vi "Average Grayscale of Line.vi"(8 "nPoints":i32, 9 "offset":i32, 10 "row":i32, 11 "24-bit pixmap in":u32[][](array[numeric])) -> (2 "average grayscale":sgl, 3 "24-bit pixmap out":u32[][](array[numeric]))   [LabVIEW 2020, in "lv_icon.lvlib"]
doc: "Find the average grayscale value along one row of a 24-bit pixmap. Uses the luminance formula:\n\nGrayscale = 0.2126 R + 0.7152 G + 0.0722 B\n\nWhere R, G, and B are the red, green, and blue intensities, respectively."
uses:
  resource/plugins/lv_icon.lvlib
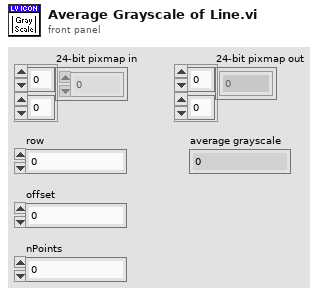
[diagram p1: front panel]
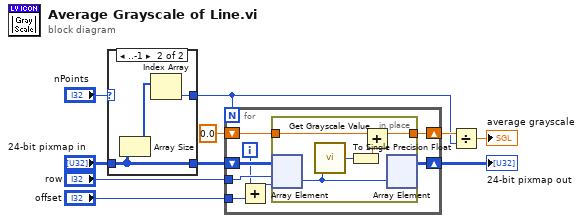
[diagram p0: block diagram]
diagram:
  n1 = case shown="..-1" "nPoints" {
    selector: "nPoints" -> [w12 _]
    tunnel: [w12 w14] -> w4
    tunnel: "24-bit pixmap in" -> [w11 w13]
    tunnel: [w11 w13] -> w2
    frame 0.. {
    }
    frame ..-1 {
      n2 = Array Size(array=w13) -> (size(s)=w15:i32[])
      n3 = Index Array(array=w15) -> (element=w14:i32)  [unwired: 1 in]
    }
  }
  n4 = for {
    N: w4 -> [_]
    tunnel: "row" -> [w22]
    shift-right: [w19] -> w9
    shift-left: sgl 0.0 ("single precision float") -> [w20]
    shift-right: [w18] -> w10
    shift-left: w2 -> [w23]
    tunnel: "offset" -> [w16]
    i -> [w17]
    n5 = Add(x=w17, y=w16) -> (x+y=w21:i32)
    n6 = in-place {
      in-place-border: w20 -> [w26]
      in-place-border: [w24] -> w19
      n7 = in-place-array #1(w23, w22, w21) -> (w28:u32)
      n8 = call "Get Grayscale Value.vi"("input color"=w28) -> ("grayscale value"=w27:u8)  [unwired: 4 in]
      n9 = To Single Precision Float(number=w27) -> (single precision float=w25:sgl)
      n10 = Add(x=w26, y=w25) -> (x+y=w24:sgl)
      n11 = in-place-array #1(w28) -> (w18:u32[][])  [unwired: 2 out]
    }
  }
  "24-bit pixmap out" <- w10
  n12 = Divide(x=w9, y=w4) -> (x/y=→"average grayscale":sgl)
